vi "TEST Dialog Dynamic.vi"() -> ()   [LabVIEW 2020, in "Multiple Errors.lvclass"]
uses:
  Multiple Errors.lvclass
panel:
  in  "Errors":i32=1
  in  "close":bool
  in  "Open if error? [T]":bool=TRUE
  in  "Open if no error? [F]":bool=TRUE
  in  "no error":bool
  out "Array":bool[](array[boolean])
  in  "error":bool
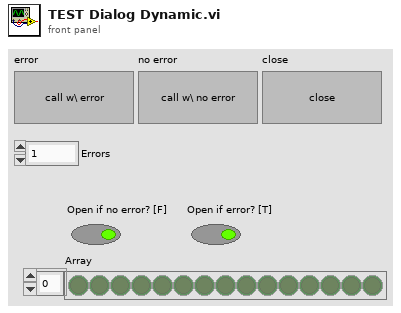
[diagram p1: front panel]
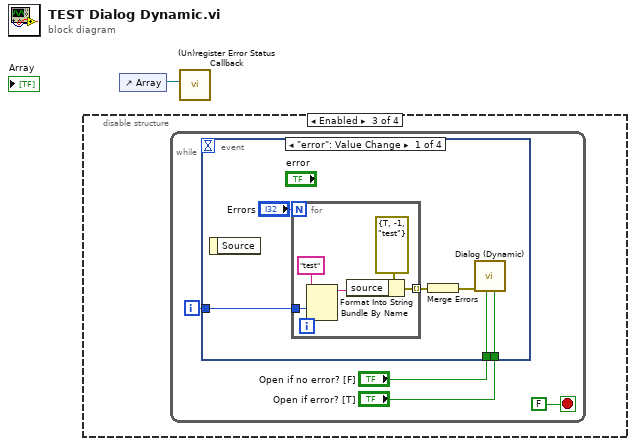
[diagram p0: block diagram]
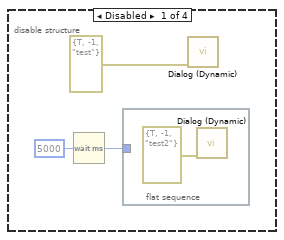
[diagram p2: hidden frame]
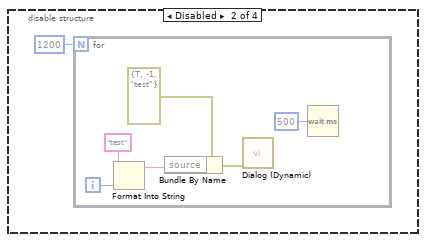
[diagram p3: hidden frame]
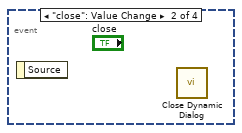
[diagram p4: hidden frame]
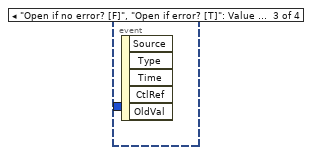
[diagram p5: hidden frame]
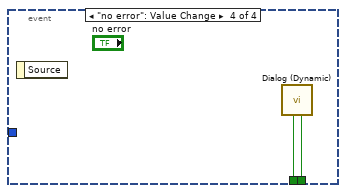
[diagram p6: hidden frame]
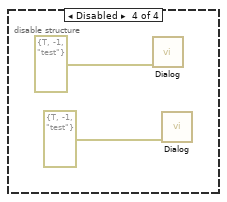
[diagram p7: hidden frame]
diagram:
  n1 = disable-structure shown="Enabled" {
    frame Disabled {
      n2 = Wait (ms)(milliseconds to wait=u32 5000) -> (millisecond timer value=w3:u32)
      n3 = flat-sequence {
        tunnel: w3 -> [_]
        frame #0 {
          n4 = call "Dialog (Dynamic).vi"("error in (no error)"=errorcluster {"status"=TRUE, "code"=-1, "source"="test2"}) -> ()  [unwired: 10 in, 1 out]
        }
      }
      n5 = call "Dialog (Dynamic).vi"("error in (no error)"=errorcluster {"status"=TRUE, "code"=-1, "source"="test"}) -> ()  [unwired: 10 in, 1 out]
    }
    frame Disabled {
      n6 = for {
        N: 1200 -> [_]
        i -> [w9]
        n7 = Format Into String(initial string="test" ("source"), w9) -> (resulting string=w7:string)  [unwired: 2 in, 1 out]
        n8 = Bundle By Name(cluster=errorcluster {"status"=TRUE, "code"=-1, "source"="test"} ("error in (no error)"), "source"=w7) -> (w10:errorcluster)
        n9 = call "Dialog (Dynamic).vi"("error in (no error)"=w10) -> ()  [unwired: 10 in, 1 out]
        n10 = Wait (ms)(milliseconds to wait=u32 500) -> ()  [unwired: 1 out]
      }
    }
    frame Enabled {
      n11 = while {
        i -> [w16]
        stop <- FALSE stop-if-true
        n12 = event shown="[0] \"error\": Value Change" {
          selector: _ -> [_ _ _ _]
          dyn-events: _ -> [_ _ _ _]
          timeout: _ -> [_ _ _ _]
          tunnel: w16 -> [w22 _ _ _]
          tunnel: "Open if no error? [F]" -> [w20 _ _ w30]
          tunnel: "Open if error? [T]" -> [w19 _ _ w29]
          event "error": Value Change {
            n13 = event-data() -> ()  [unwired: 1 in, 1 out]
            n14 = for {
              N: "Errors" -> [_]
              tunnel: w22 -> [w27]
              tunnel: [w24] -> w21 mode=indexing
              i -> [w23]
              n15 = Format Into String(initial string="test" ("source"), w27, w23) -> (resulting string=w25:string)  [unwired: 2 in, 1 out]
              n16 = Bundle By Name(cluster=errorcluster {"status"=TRUE, "code"=-1, "source"="test"} ("error in (no error)"), "source"=w25) -> (w24:errorcluster)
            }
            n17 = Merge Errors(w21) -> (w18:errorcluster)
            n18 = call "Dialog (Dynamic).vi"("Open if error? [T]"=w19, "Open if no error? [F]"=w20, "error in (no error)"=w18) -> ()  [unwired: 8 in, 1 out]
          }
          event "close": Value Change {
            n19 = event-data() -> ()  [unwired: 1 in, 1 out]
            n20 = call "Close Dynamic Dialog.vi"() -> ()  [unwired: 11 in, 1 out]
          }
          event "Open if no error? [F]", "Open if error? [T]": Value Change {
            n21 = event-data() -> ()  [unwired: 1 in, 5 out]
          }
          event "no error": Value Change {
            n22 = event-data() -> ()  [unwired: 1 in, 1 out]
            n23 = call "Dialog (Dynamic).vi"("Open if error? [T]"=w29, "Open if no error? [F]"=w30) -> ()  [unwired: 9 in, 1 out]
          }
        }
      }
    }
    frame Disabled {
      n24 = call "Dialog.vi"("error in (no error)"=errorcluster {"status"=TRUE, "code"=-1, "source"="test"}) -> ()  [unwired: 11 in]
      n25 = call "Dialog.vi"("error in (no error)"=errorcluster {"status"=TRUE, "code"=-1, "source"="test"}) -> ()  [unwired: 11 in]
    }
  }
  n26 = control-ref of="Array"() -> (w1:refnum<vi>)
  n27 = call "(Un)register Error Status Callback.vi"("Arr Refnum [NOP]"=w1) -> ()  [unwired: 10 in, 1 out]
